vi "TraverseControl_High.vi"(0 "Mode":T1=enum."Read traverse position", 1 "Route Checking?":bool, 3 "Traverse Name":string, 7 "Model       Roll      Pitch       Yaw (deg)":dbl[](array[numeric]) format="%#.2f", 11 "Position input XYZ":dbl[](array[numeric])=[0.0, 0.0, 0.0] format="%.2f", 12 "Last Part of Move?":bool, 13 "Speed Factor":dbl=1.0 min=0.1 max=5.0 format="%.2f", 14 "Backlash Compensation?":bool=TRUE) -> (4 "Position Output XYZ":dbl[](array[numeric]) format="%.2f", 15 "Error String":string)   [LabVIEW 2013]
uses:
  Anemometry/Anemometry Sub Vis/Gen Trav/Trav_mode.ctl
  Anemometry/Anemometry Sub Vis/Globals/Trav_pos_global.vi
  Anemometry/Anemometry Sub Vis/Gen Trav/Route mapping/Route_mapping_global.vi
  Anemometry/Anemometry Sub Vis/Globals/Preference_global.vi
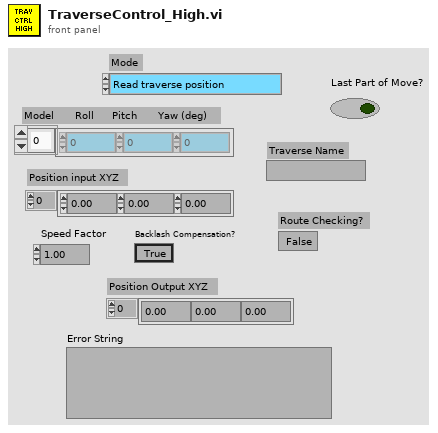
[diagram p1: front panel]
types:
  T1 = typedef "Trav_mode.ctl" = enum16{"Move traverse", "Read traverse position", "Teach Position"}
  T2 = typedef "Tunnel_Coordinates.ctl" = enum16{"Work in Tunnel Coordinates", "Work in Model Coordinates"}
  T3 = typedef "Box_size.ctl" = cluster{"Max":dbl, "Min":dbl}[]
  T4 = typedef "Exclude_cluster.ctl" = cluster{"Sizes":T3, "Name":string, "Exclude Type":T5}
  T5 = typedef "Exclusion_type.ctl" = enum16{"Exclude completely", "Allow only vertical moves"}
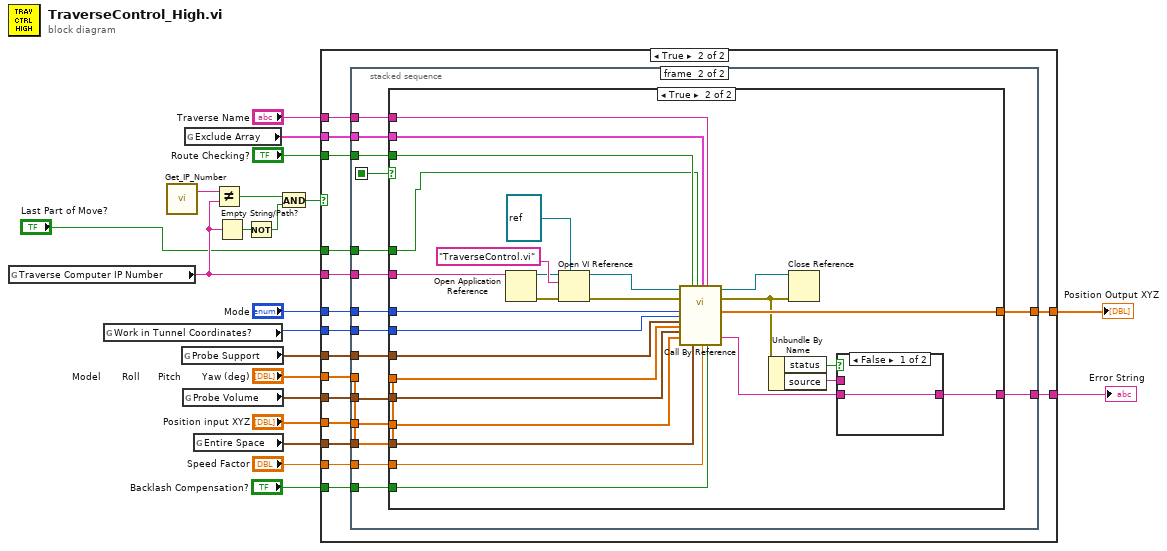
[diagram p0: block diagram]
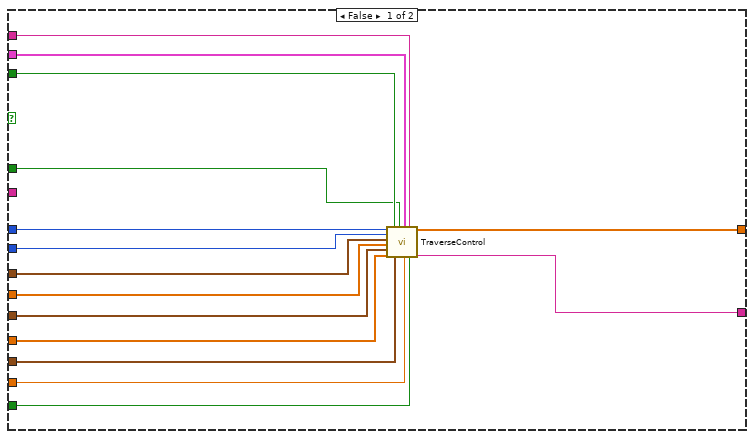
[diagram p2: hidden frame]
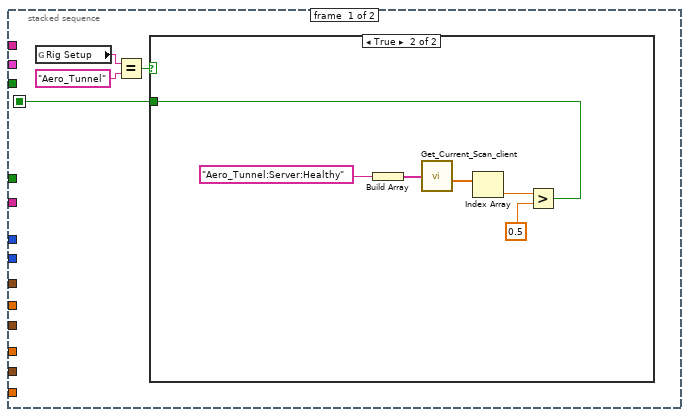
[diagram p3: hidden frame]
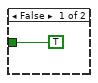
[diagram p4: hidden frame]
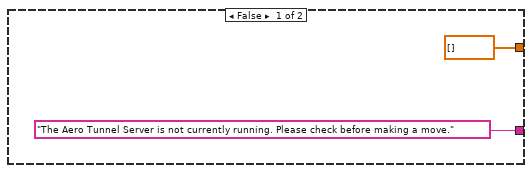
[diagram p5: hidden frame]
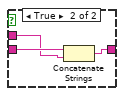
[diagram p6: hidden frame]
diagram:
  n1 = global read "Trav_pos_global.vi" "Traverse Computer IP Number"() -> (w9:string)
  n2 = global read "Trav_pos_global.vi" "Work in Tunnel Coordinates?"() -> (w3:T2)
  n3 = call "Get_IP_Number.vi"() -> ("IP Number"=w21:string)  [unwired: 1 out]
  n4 = global read "Route_mapping_global.vi" "Probe Support"() -> (w2:T3)
  n5 = global read "Route_mapping_global.vi" "Probe Volume"() -> (w4:T3)
  n6 = global read "Route_mapping_global.vi" "Exclude Array"() -> (w6:T4[])
  n7 = global read "Route_mapping_global.vi" "Entire Space"() -> (w5:T3)
  n8 = Not Equal?(x=w21, y=w9) -> (x != y?=w8:bool)
  n9 = Empty String/Path?(string/path=w9) -> (empty?=w11:bool)
  n10 = Not(x=w11) -> (.not. x?=w10:bool)
  n11 = And(x=w8, y=w10) -> (x .and. y?=w7:bool)
  n12 = case shown="True" w7 {
    tunnel: "Route Checking?" -> [w29 w52]
    tunnel: "Traverse Name" -> [w28 w51]
    tunnel: [w35 w50] -> w18
    tunnel: [w36 w42] -> w17
    tunnel: "Backlash Compensation?" -> [w32 w49]
    tunnel: "Speed Factor" -> [w31 w48]
    tunnel: "Position input XYZ" -> [w34 w47]
    tunnel: "Model       Roll      Pitch       Yaw (deg)" -> [w33 w46]
    tunnel: "Mode" -> [w30 w45]
    tunnel: w9 -> [_ w44]
    tunnel: w6 -> [w27 w43]
    tunnel: w5 -> [w26 w39]
    tunnel: w4 -> [w25 w40]
    tunnel: w3 -> [w24 w41]
    tunnel: w2 -> [w23 w38]
    tunnel: "Last Part of Move?" -> [w22 w37]
    frame False {
      n13 = call "TraverseControl.vi"("Mode"=w30, "Work in Tunnel Coordinates?"=w24, "Probe Support"=w23, "Model       Roll      Pitch       Yaw (deg)"=w33, "Probe Volume"=w25, "Position input XYZ"=w34, "Route Checking?"=w29, "Entire Space"=w26, "Last Part of Move?"=w22, "Exclude Array"=w27, "Speed Factor"=w31, "Traverse Name"=w28, "Backlash Compensation?"=w32) -> ("Position Output XYZ"=w35:dbl[], "Error String"=w36:string)  [unwired: 5 in]
    }
    frame True {
      n14 = stacked-sequence {
        seq-local: [w53 _] -> [_ w66]
        tunnel: w52 -> [_ w80]
        tunnel: w51 -> [_ w79]
        tunnel: [_ w78] -> w50
        tunnel: w49 -> [_ w77]
        tunnel: w48 -> [_ w76]
        tunnel: w47 -> [_ w75]
        tunnel: w46 -> [_ w74]
        tunnel: w45 -> [_ w73]
        tunnel: w44 -> [_ w72]
        tunnel: w43 -> [_ w71]
        tunnel: [_ w70] -> w42
        tunnel: w41 -> [_ w69]
        tunnel: w40 -> [_ w68]
        tunnel: w39 -> [_ w67]
        tunnel: w38 -> [_ w65]
        tunnel: w37 -> [_ w64]
        frame #0 {
          n15 = global read "Preference_global.vi" "Rig Setup"() -> (w56:string)
          n16 = Equal?(x=w56, y="Aero_Tunnel" ("Rig Setup")) -> (x = y?=w54:bool)
          n17 = case shown="True" w54 {
            tunnel: [TRUE w58] -> w53
            frame False {
            }
            frame True {
              n18 = Build Array("Aero_Tunnel:Server:Healthy") -> (w63:string[])
              n19 = call "Get_Current_Scan_client.vi"("ADAM Ch Names"=w63) -> ("Numerical Values"=w61:dbl[])  [unwired: 3 out]
              n20 = Index Array(array=w61) -> (element=w60:dbl)  [unwired: 1 in]
              n21 = Greater?(x=w60, y=0.5) -> (0:w58:bool)
            }
          }
        }
        frame #1 {
          n22 = case shown="True" w66 {
            tunnel: w80 -> [_ w106]
            tunnel: w79 -> [_ w105]
            tunnel: [dbl[] [] ("Position Output XYZ") w104] -> w78
            tunnel: w77 -> [_ w103]
            tunnel: w76 -> [_ w102]
            tunnel: w75 -> [_ w101]
            tunnel: w74 -> [_ w100]
            tunnel: w73 -> [_ w99]
            tunnel: w72 -> [_ w96]
            tunnel: w71 -> [_ w93]
            tunnel: ["The Aero Tunnel Server is not currently running. Please check before making a move." ("Error String") w90] -> w70
            tunnel: w69 -> [_ w87]
            tunnel: w68 -> [_ w86]
            tunnel: w67 -> [_ w85]
            tunnel: w65 -> [_ w84]
            tunnel: w64 -> [_ w83]
            frame False {
            }
            frame True {
              n23 = Open Application Reference(11:w96) -> (0:w94:errorcluster, 3:w95:refnum<vi>)  [unwired: 2 in, 1 out]
              n24 = Open VI Reference(type specifier VI Refnum (for type only)=refnum<vi> refnum ("Scout Server"), application reference (local)=w95, vi path="TraverseControl.vi", error in (no error)=w94) -> (vi reference=w107:refnum<vi>, error out=w98:errorcluster)  [unwired: 2 out]
              n25 = call-by-ref "?"(reference=w107, error in=w98, "Mode"=w99, "Work in Tunnel Coordinates?"=w87, "Probe Support"=w84, "Model       Roll      Pitch       Yaw (deg)"=w100, "Probe Volume"=w86, "Position input XYZ"=w101, "Route Checking?"=w106, "Entire Space"=w85, "Last Part of Move?"=w83, "Exclude Array"=w93, "Speed Factor"=w102, "Traverse Name"=w105, "Backlash Compensation?"=w103) -> (reference out=w97:refnum<vi>, error out=w92:errorcluster, "Position Output XYZ"=w104:dbl[], "Error String"=w89:string)  [unwired: 5 in]
              n26 = Unbundle By Name(w92) -> ("status"=w91:bool, "source"=w88:string)
              n27 = Close Reference(reference=w97, error in (no error)=w92) -> ()  [unwired: 1 out]
              n28 = case shown="False" w91 {
                tunnel: [w110 w113] -> w90
                tunnel: w89 -> [w110 w112]
                tunnel: w88 -> [_ w111]
                frame False {
                }
                frame True {
                  n29 = Concatenate Strings(w112, w111) -> (w113:string)
                }
              }
            }
          }
        }
      }
    }
  }
  "Error String" <- w17
  "Position Output XYZ" <- w18
